vi "Datasheet Generate Run Summary.vi"(7 "Connection Refnum":T1, 8 "error in (no error)":errorcluster, 11 "File Information":T2) -> (0 "error out":errorcluster, 3 "Summary File Path":path)   [LabVIEW 2011]
uses:
  TDMS/TDMS File.ctl
  TDMS/TDMS Run.ctl
  TDMS/TDMS Channel (Sxx).ctl
  database/Fields/Field Record.ctl
  database/Fields/Field DataTypes.ctl
  database/Fields/Field NextItem.ctl
  Summitek EXT/ODBC/SQL Controls/Connection Refnum.ctl
panel:
  out "concatenated string":string
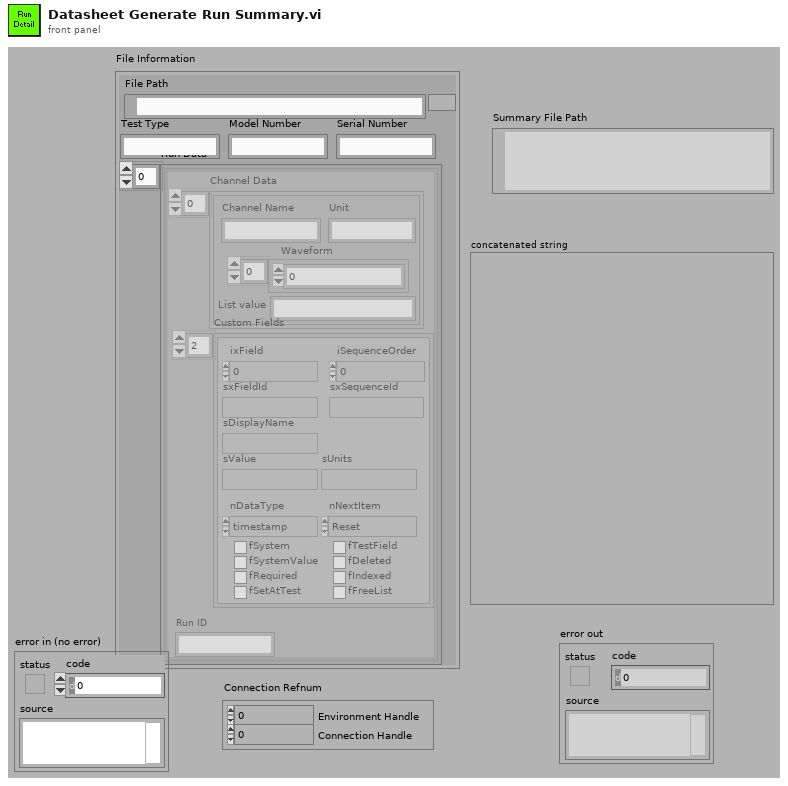
[diagram p1: front panel]
types:
  T1 = typedef "Connection Refnum.ctl" = cluster{"Environment Handle":i32, "Connection Handle":i32}
  T2 = typedef "TDMS File.ctl" = cluster{"File Path":path, "Run Data":T3[], "Serial Number":string, "Model Number":string, "Test Type":string}
  T3 = typedef "TDMS Run.ctl" = cluster{"Channel Data":T4[], "Custom Fields":T5[], "Run ID":string}
  T4 = typedef "TDMS Channel (Sxx).ctl" = cluster{"Channel Name":string, "Waveform":dbl[], "Unit":string, "List value":string}
  T5 = typedef "Field Record.ctl" = cluster{"ixField":i32, "iSequenceOrder":i32, "sxFieldId":string, "sxSequenceId":string, "sDisplayName":string, "sValue":string, "sUnits":string, "nDataType":T6, "nNextItem":T7, "fSystem":bool, "fSystemValue":bool, "fRequired":bool, "fSetAtTest":bool, "fTestField":bool, "fDeleted":bool, "fIndexed":bool, "fFreeList":bool}
  T6 = typedef "Field DataTypes.ctl" = enum32{"text", "numeric", "list", "timestamp", "boolean"}
  T7 = typedef "Field NextItem.ctl" = enum32{"Reset", "Retain", "Auto-Increment"}
  T8 = enum16{"open", "replace", "create", "open or create", "replace or create", "replace or create with confirmation"}
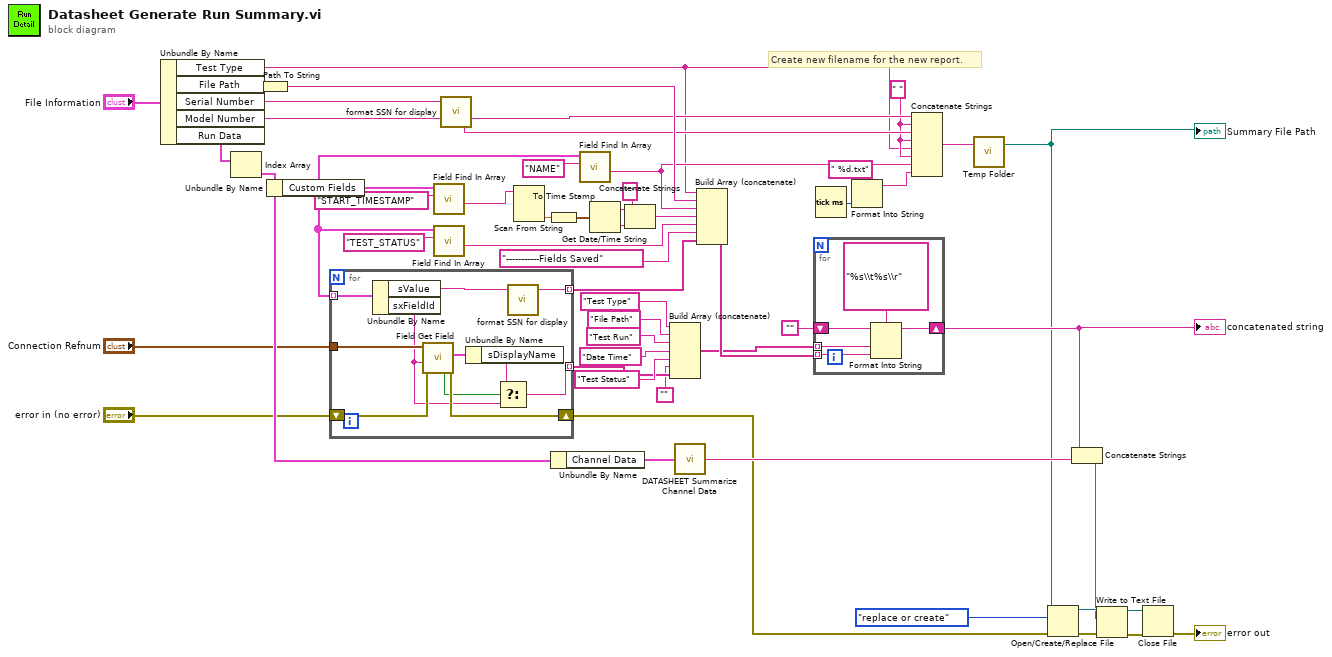
[diagram p0: block diagram]
diagram:
  w5 = " " ("regular expression")
  # "Create new filename for the new report."
  n1 = Unbundle By Name("File Information") -> ("Test Type"=w4:string, "File Path"=w41:path, "Serial Number"=w25:string, "Model Number"=w7:string, "Run Data"=w49:T3[])
  n2 = Index Array(array=w49) -> (element=w27:T3)  [unwired: 1 in]
  n3 = Path To String(path=w41) -> (string=w40:string)
  n4 = Unbundle By Name(w27) -> ("Custom Fields"=w20:T5[])
  n5 = for {
    tunnel: w20 -> [w64] mode=indexing
    tunnel: [w62] -> w42 mode=indexing
    tunnel: "Connection Refnum" -> [w61]
    tunnel: [w55] -> w11 mode=indexing
    shift-right: [w58] -> w3
    shift-left: "error in (no error)" -> [w59]
    n6 = Unbundle By Name(w64) -> ("sValue"=w63:string, "sxFieldId"=w54:string)
    n7 = call "Field Get Field.vi"("error in (no error)"=w59, "sFieldId or sDisplayName (\"\")"=w54, "Connection Refnum"=w61) -> ("error out"=w58:errorcluster, "Field"=w60:T5, "Data Present?"=w57:bool)  [unwired: 2 in, 4 out]
    n8 = Unbundle By Name(w60) -> ("sDisplayName"=w56:string)
    n9 = Select(t=w56, s=w57, f=w54) -> (s? t:f=w55:string)
    n10 = call "format SSN for display.vi"("string"=w63) -> ("s? t:f"=w62:string)  [unwired: 4 out]
  }
  n11 = call "Field Find In Array.vi"("FieldID or Display Name(\"\")"="START_TIMESTAMP" ("format string"), "Field Array"=w20) -> ("sValue"=w17:string)  [unwired: 1 in, 8 out]
  n12 = call "Field Find In Array.vi"("FieldID or Display Name(\"\")"="TEST_STATUS" ("format string"), "Field Array"=w20) -> ("sValue"=w16:string)  [unwired: 1 in, 8 out]
  n13 = call "format SSN for display.vi"("string"=w25) -> ("s? t:f"=w6:string)  [unwired: 4 out]
  n14 = Scan From String(input string=w17) -> (output 1=w18:dbl)  [unwired: 3 in, 4 out]
  n15 = To Time Stamp(1:w18) -> (0:w19:timestamp)
  n16 = Unbundle By Name(w27) -> ("Channel Data"=w26:T4[])
  n17 = call "Field Find In Array.vi"("FieldID or Display Name(\"\")"="NAME" ("format string"), "Field Array"=w20) -> ("sValue"=w23:string)  [unwired: 1 in, 8 out]
  n18 = Get Date/Time String(seconds (now)=w19) -> (date string=w39:string, time string=w38:string)  [unwired: 2 out]
  n19 = Concatenate Strings(w39, " " ("regular expression"), w38) -> (w36:string)
  n20 = Build Array (concatenate)("Test Type" ("format string"), "File Path" ("format string"), "Test Run" ("format string"), "Date Time" ("format string"), "Test Status" ("format string"), "", w11) -> (w34:string[])
  n21 = call "DATASHEET Summarize Channel Data.vi"("Channel Data"=w26) -> ("HTM Table Rows"=w15:string)
  n22 = Build Array (concatenate)(w4, w40, w23, w36, w16, "-----------Fields Saved" ("format string"), w42) -> (w35:string[])
  n23 = for {
    shift-right: [w68] -> w13
    shift-left: "" -> [w67]
    tunnel: w35 -> [w66] mode=indexing
    tunnel: w34 -> [w65] mode=indexing
    n24 = Format Into String(format string="%s\\t%s\\r", initial string=w67, w65, w66) -> (resulting string=w68:string)  [unwired: 1 in, 1 out]
  }
  "concatenated string" <- w13
  n25 = Tick Count (ms)() -> (millisecond timer value=w52:u32)
  n26 = Format Into String(format string=" %d.txt", w52) -> (resulting string=w53:string)  [unwired: 2 in, 1 out]
  n27 = Concatenate Strings(w7, w5, w6, w5, w4, w5, w23, w53) -> (w2:string)
  n28 = call "Temp Folder.vi"("Relative Path (\"\")"=w2) -> ("Temp Folder"=w1:path)  [unwired: 2 in]
  "Summary File Path" <- w1
  n29 = Open/Create/Replace File(file path (use dialog)=w1, error in=w3, operation (0:open)=T8."replace or create") -> (refnum out=w47:refnum<file>, error out=w46:errorcluster)  [unwired: 4 out]
  n30 = Concatenate Strings(w13, w15) -> (w14:string)
  n31 = Write to Text File(file (use dialog)=w47, text=w14, error in=w46) -> (refnum out=w45:refnum<file>, error out=w44:errorcluster)  [unwired: 2 out]
  n32 = Close File(refnum=w45, error in=w44) -> (error out=→"error out":errorcluster)  [unwired: 1 out]
